vi "填充树形控件基本方法.vi"() -> ()   [LabVIEW 2012, in "Tree Tools.lvlib"]
uses:
  Tree Tools.lvlib
  Core Class/Tree Class/Tree Class.lvclass
panel:
  out "标识符":string
  in  "布尔":bool
  out "error out":errorcluster
  in  "Tree":string(tree)
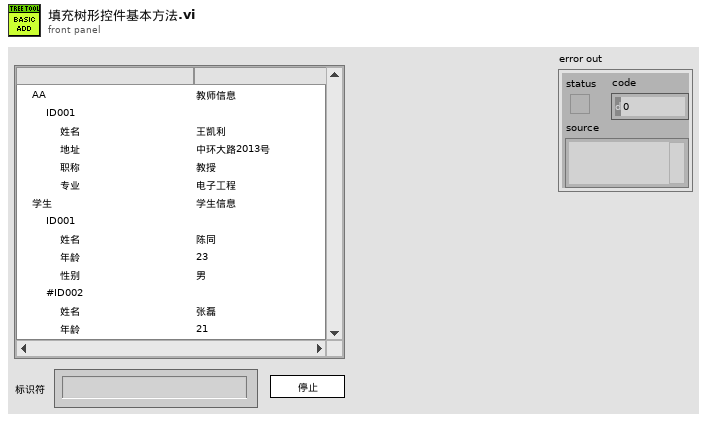
[diagram p1: front panel]
types:
  T1 = cluster{"姓名":string, "年龄":u8, "性别":enum16{"男", "女"}}
  T2 = cluster{"姓名":string, "地址":string, "职称":enum16{"教授", "副教授", "讲师"}, "专业":enum16{"工业自动化", "电子工程"}}
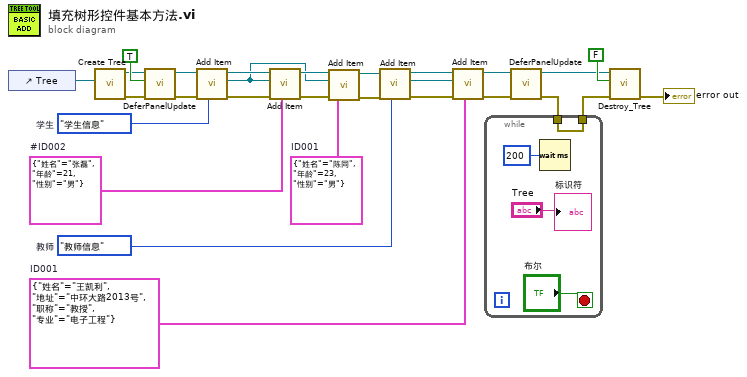
[diagram p0: block diagram]
diagram:
  w3 = T1 {"姓名"="陈同", "年龄"=23, "性别"=enum."男"}  # ID001
  w9 = enum16{"学生信息", "教师信息"}."教师信息"  # 教师
  w18 = T2 {"姓名"="王凯利", "地址"="中环大路2013号", "职称"=enum."教授", "专业"=enum."电子工程"}  # ID001
  w19 = T1 {"姓名"="张磊", "年龄"=21, "性别"=enum."男"}  # #ID002
  w27 = enum16{"学生信息", "教师信息"}."学生信息"  # 学生
  n1 = control-ref of="Tree"() -> (w28:refnum<vi>)
  n2 = call "Create Tree.vi"("Tree Refnum"=w28) -> ("error out"=w14:errorcluster, "Tree_LVOOP out"=w16:refnum<class "Tree Class.lvclass">)  [unwired: 2 in, 7 out]
  n3 = call-dynamic "DeferPanelUpdate.vi"("error in (no error)"=w14, "Defer? (F)"=TRUE, "Tree_LVOOP__lava_lib_tree_class in"=w16) -> ("error out"=w13:errorcluster, "Tree_LVOOP__lava_lib_tree_class out"=w15:refnum<class "Tree Class.lvclass">)  [unwired: 7 in]
  n4 = call-dynamic "Add Item.vi"("Data"=w27, "error in (no error)"=w13, "Tree_LVOOP in"=w15) -> ("error out"=w23:errorcluster, "Upmost Created Tag"=w4:refnum<class "Tree Tag Class.lvclass">, "Tree_LVOOP out"=w26:refnum<class "Tree Class.lvclass">)  [unwired: 6 in]
  n5 = call-dynamic "Add Item.vi"("Data"=w19, "error in (no error)"=w23, "Parent Tag"=w4, "Tree_LVOOP in"=w26) -> ("error out"=w7:errorcluster, "Tree_LVOOP out"=w8:refnum<class "Tree Class.lvclass">)  [unwired: 5 in, 1 out]
  n6 = call-dynamic "Add Item.vi"("Data"=w3, "error in (no error)"=w7, "Parent Tag"=w4, "Tree_LVOOP in"=w8) -> ("error out"=w5:errorcluster, "Tree_LVOOP out"=w6:refnum<class "Tree Class.lvclass">)  [unwired: 5 in, 1 out]
  n7 = call-dynamic "Add Item.vi"("Data"=w9, "error in (no error)"=w5, "Tree_LVOOP in"=w6) -> ("error out"=w22:errorcluster, "Upmost Created Tag"=w25:refnum<class "Tree Tag Class.lvclass">, "Tree_LVOOP out"=w24:refnum<class "Tree Class.lvclass">)  [unwired: 6 in]
  n8 = call-dynamic "Add Item.vi"("Data"=w18, "error in (no error)"=w22, "Parent Tag"=w25, "Tree_LVOOP in"=w24) -> ("error out"=w12:errorcluster, "Tree_LVOOP out"=w11:refnum<class "Tree Class.lvclass">)  [unwired: 5 in, 1 out]
  n9 = call-dynamic "DeferPanelUpdate.vi"("error in (no error)"=w12, "Tree_LVOOP__lava_lib_tree_class in"=w11) -> ("error out"=w2:errorcluster, "Tree_LVOOP__lava_lib_tree_class out"=w10:refnum<class "Tree Class.lvclass">)  [unwired: 8 in]
  n10 = while {
    tunnel: w2 -> [w29]
    tunnel: [w29] -> w1
    stop <- "布尔" stop-if-true
    n11 = Wait (ms)(milliseconds to wait=u32 200 ("等待时间（毫秒）")) -> ()  [unwired: 1 out]
    "标识符" <- "Tree"
  }
  n12 = call-dynamic "Destroy_Tree.vi"("error in (no error)"=w1, "Delete Tree Items? (F)"=FALSE, "Tree_LVOOP in"=w10) -> ("error out"=→"error out":errorcluster)  [unwired: 8 in]
